vi "FRIC_navX_Internal_USB_ProcessingLoop.vi"(7 "Device Number":T3, 10 "Serial Port":T2=enum."USB 1", 11 "Rate (4Hz-200Hz)":u8=50 min=4 max=200) -> ()   [LabVIEW 2025]
doc: "This navX VI handles the reading/writing for the navX. All of the good stuff is in here.\nTHIS VI SHOULD NOT BE CALLED BY THE USER!"
uses:
  _TypeDefs/Z900_navX_SerialStreamTypeDef.ctl
  _TypeDefs/FRIC_navX_DeviceNumbersTypeDef.ctl
  <vilib>/Rock Robotics/WPI/SerialPort/WPI_SerialPort.ctl
  _TypeDefs/Z900_navX_ProtocolTypeDef.ctl
  _TypeDefs/FRIC_navX_ProcessingLoopStatesTypeDef_I2C.ctl
  _TypeDefs/FRIC_navX_I2C Process Loop TypeDef.ctl
  _TypeDefs/Z900_navX_DeviceTypeDef.ctl
  _TypeDefs/Z900_navX_NotifyPacketTypeDef.ctl
  _TypeDefs/Z900_navX_ActionTypeDef.ctl
  <vilib>/Rock Robotics/SystemInterfaces/i2clib/i2c_bus.ctl
  _TypeDefs/Z900_navX_IntegrationControlRegisters.ctl
  <vilib>/Rock Robotics/WPI/SPI/WPI_SPIDevRef.ctl
  <vilib>/Rock Robotics/SystemInterfaces/spilib/spi_bus.ctl
  <vilib>/Rock Robotics/WPI/SerialPort/WPI_SerialPortRef.ctl
  <vilib>/Platform/TimedLoop/XDataNode/timing_clust.ctl
  <vilib>/Platform/TimedLoop/XDataNode/nitl_modes.ctl
  <vilib>/Platform/TimedLoop/XDataNode/wakeup.ctl
  <vilib>/Rock Robotics/SystemInterfaces/NetworkCommunication/NetComm_UsageReport_ResourceType.ctl
  <vilib>/Rock Robotics/SystemInterfaces/Utilities/FPGA_UtilitiesRead LocalTime.vi
  <vilib>/Platform/TimedLoop/XDataNode/XDataNode.xnode
  <vilib>/Platform/TimedLoop/XDataNode/XDNodeRunTimeDep.lvlib
panel:
  in  "Tab Control":enum32{"Page 1", "Page 2"}(tab)
  in  "Halt":bool
  out "Connected 2":bool
  out "error":errorcluster
  in  "Stream Type":T1=enum."AHRSAndPositioning"
  out "Loop TIme":i64
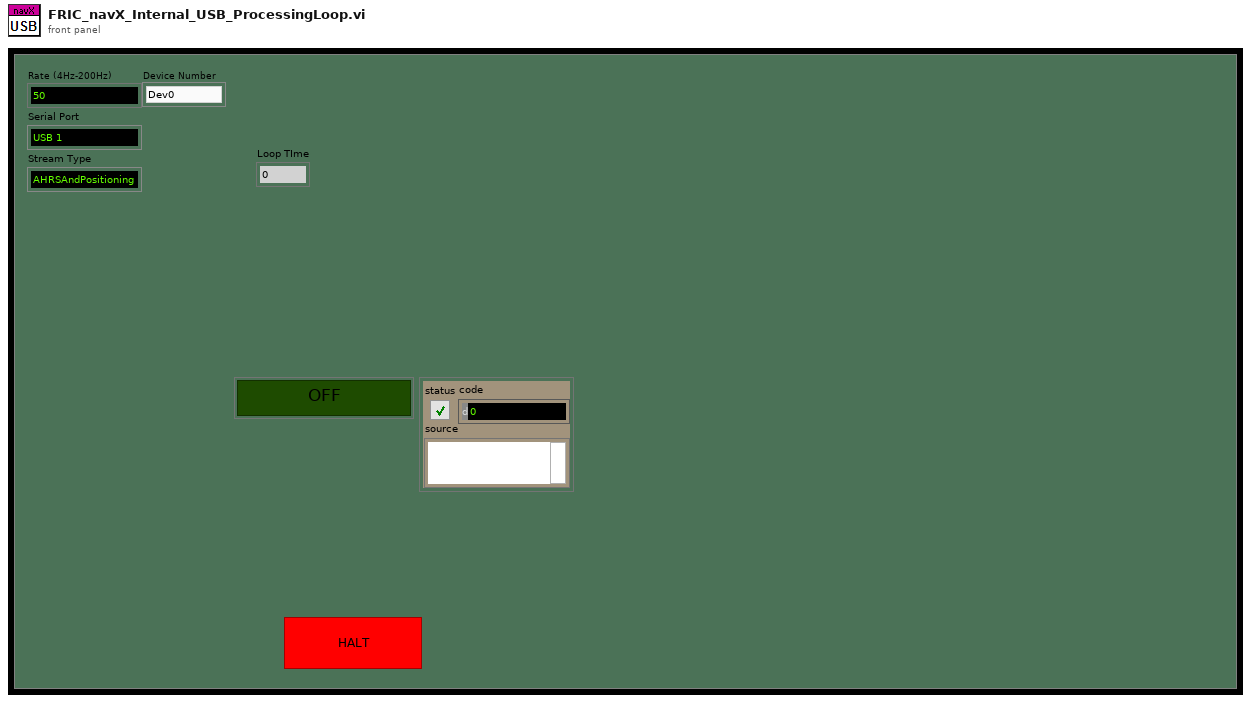
[diagram p1: front panel]
types:
  T1 = typedef "Z900_navX_SerialStreamTypeDef.ctl" = enum16{"YRPH", "Quaterinons", "Gyro/Raw", "AHRS", "AHRSAndPositioning", "AHRSAndPOSTime"}
  T2 = typedef "WPI_SerialPort.ctl" = enum16{"Onboard RS-232", "MXP TTL", "USB 1", "USB 2"}
  T3 = typedef "FRIC_navX_DeviceNumbersTypeDef.ctl" = enum16{"Dev0", "Dev1", "Dev2", "Dev3"}
  T4 = typedef "FRIC_navX_I2C Process Loop TypeDef.ctl" = cluster{"State Array":T5[], "error":errorcluster, "FPGA Cluster":cluster{"Last Valid FPGA Time":dbl, "Error Count":i32, "Initialized":bool}, "Device Info":T6, "I2CDevRef":cluster{"DevStatus":errorcluster, "Device Address":u8, "Handle":i32, "I2C Bus":T8}, "Registry":u8[], "Command Array":T9[], "Connected?":bool, "navX Device Memory Size":i32, "notification":T10, "Memory Size Set":bool, "SPIDevRef":T12, "navX Serial Open":cluster{"Stream Type":T1, "Serial Port":T2}, "SerialPortRef":T14, "Serial Read Buffer":string, "Serial Write Buffer":string[], "Device Number":T3, "navX SPI Open":cluster{"SPI Bus":T13, "Clock Rate (Hz)":dbl}, "Loop dt":i64, "current time":timestamp, "Loop Time":i64}
  T5 = typedef "FRIC_navX_ProcessingLoopStatesTypeDef_I2C.ctl" = enum16{"Process", "INI", "Check Packets Valid", "Close", "Clear VISA", "Generate Command", "Last Packet Valid", "Open", "Read", "Reset Serial", "Set Termination Char", "Update AE", "Wait", "Write", "Exit"}
  T6 = typedef "Z900_navX_DeviceTypeDef.ctl" = cluster{"Interface":cluster{"Protocol":T7, "Update Rate (4Hz-200Hz)":u8, "navX Open TypeDef":variant}, "Notify Packet":refnum<notifier>, "Loop VI Refnum":refnum<vi>, "Ready to Close Occurrence Refnum":refnum<k4>, "Name":string}
  T7 = typedef "Z900_navX_ProtocolTypeDef.ctl" = enum16{"SERIAL", "I2C", "SPI"}
  T8 = typedef "i2c_bus.ctl" = enum16{"I2C On-Board", "I2C MXP", "Invalid"}
  T9 = typedef "Z900_navX_IntegrationControlRegisters.ctl" = u8
  T10 = typedef "Z900_navX_NotifyPacketTypeDef.ctl" = cluster{"navX Action":T11, "Data":variant, "Stream Type":T1, "Device Number":T3}
  T11 = typedef "Z900_navX_ActionTypeDef.ctl" = enum16{"None", "Halt", "Normal Read", "Update Serial Protocol", "Update Rate Htz", "Zero-Yaw", "Zero-Displacement", "Zero-Velocity"}
  T12 = typedef "WPI_SPIDevRef.ctl" = cluster{"DevStatus":errorcluster, "Handle":i32, "SPI Bus":T13}
  T13 = typedef "spi_bus.ctl" = enum16{"SPI On-Board, CS0", "SPI On-Board, CS1", "SPI On-Board, CS2", "SPI On-Board, CS3", "SPI MXP", "Invalid"}
  T14 = typedef "WPI_SerialPortRef.ctl" = cluster{"DevStatus":errorcluster, "Serial Port Name":refnum<visa-resource-name>}
  T15 = typedef "XDNodeRunTimeDep.lvlib/timing_clust.ctl" = cluster{"Expected End [f-1]":u64, "Actual End [f-1]":u64, "Finished Late? [f-1]":bool, "Expected End [i-1]":u64, "Actual End [i-1]":u64, "Finished Late? [i-1]":bool, "Expected Start [i]":u64, "Actual Start [i]":u64, "Expected Start [f]":u64, "Actual Start [f]":u64, "Source Name":string, "Structure Name":string, "Period":i64, "Deadline":i64, "Offset":i64, "Start":i64, "Priority":i32, "Timeout":i32, "Mode":T16, "Wakeup Reason":T17, "Error":errorcluster, "Source Type":string, "Secondary Source Type":string, "Global End Time":u64, "Global Start Time":u64, "Frame Duration":u64, "Iteration Duration":u64, "Assigned CPU":i32, "I/O Scan Engine Mode":u32}
  T16 = typedef "XDNodeRunTimeDep.lvlib/nitl_modes.ctl" = enum32{"No Change", "Process missed periods, maintain original phase", "Discard missed periods, maintain original phase", "Process missed periods, ignore original phase", "Discard missed periods, ignore original phase"}
  T17 = typedef "XDNodeRunTimeDep.lvlib/wakeup.ctl" = enum32{"Normal", "Aborted", "Asynchronous wakeup", "Timing source error", "Timed loop error", "Timeout"}
  T18 = typedef "NetComm_UsageReport_ResourceType.ctl" = enum8{"Controller", "Module", "Language", "CANPlugin", "Accelerometer", "ADXL345", "AnalogChannel", "AnalogTrigger", "AnalogTriggerOutput", "CANJaguar", "Compressor", "Counter", "Dashboard", "DigitalInput", "DigitalOutput", "DriverStationCIO", "DriverStationEIO", "DriverStationLCD", "Encoder", "GearTooth", "Gyro", "I2C", "Framework", "Jaguar", "Joystick", "Kinect", "KinectStick", "PIDController", "Preferences", "PWM", "Relay", "RobotDrive", "SerialPort", "Servo", "Solenoid", "SPI", "Task", "Ultrasonic", "Victor", "Button", "Command", "AxisCamera", "PCVideoServer", "SmartDashboard", "Talon", "HiTechnicColorSensor", "HiTechnicAccel", "HiTechnicCompass", "SRF08", "AnalogOutput", "Victor SP", "Talon SRX", "CAN Talon SRX", "ADXL362 Accel", "ADXRS450 Gyro", "Rev SPARK", "Mindsensors SD540", "Digital Filter", "ADIS16448", "PDP", "PCM", "PigeonIMU", "Nidec Brushless", "CTRE CANifier", "CTRE TalonFX", "CTRE Future 1", "CTRE Future 2", "CTRE Future 3", "CTRE Future 4", "CTRE Future 5", "CTRE Future 6", "Linear Filter", "Xbox Controller", "USB Camera", "NavX", "Pixy", "Pixy2", "ScanseSweep", "Shuffleboard", "CAN", "Digilent DMC60", "PWM Victor SPX", "Rev SPARK MAX PWM", "Rev SPARK MAX CAN", "ADIS16470", "PIDController2", "ProfiledPIDController", "Kinematics", "Odometry", "Units", "Trapezoid Profile", "DutyCycle", "Addressable LEDs", "Fusion Venom", "CTRE Future 7", "CTRE Future 8", "CTRE Future 9", "CTRE Future 10", "CTRE Future 11", "CTRE Future 12", "CTRE Future 13", "CTRE Future 14", "Exponential Profile", "PS4 Controller", "Photon Camera", "Photon Pose Estimator", "Path Planner Path", "Path Planner Auto", "Path Finding Command", "Redux Future 1", "Redux Future 2", "Redux Future 3", "Redux Future 4", "Redux Future 5", "Rev SPARK Flex CAN", "Rev SPARK Flex PWM", "LEDPattern", "LinearQuadraticRegulator", "KalmanFilter", "PoseEstimator", "PoseEstimator3d", "LinearSystemLoop", "WPILib_future7", "WPILib_future8", "Rev_ServoHub", "YAMS", "LumenLabs_ConnectorX", "LumenLabs_ConnectorXLED"}
  T19 = cluster{"Last Valid FPGA Time":dbl, "Error Count":i32, "Initialized":bool}
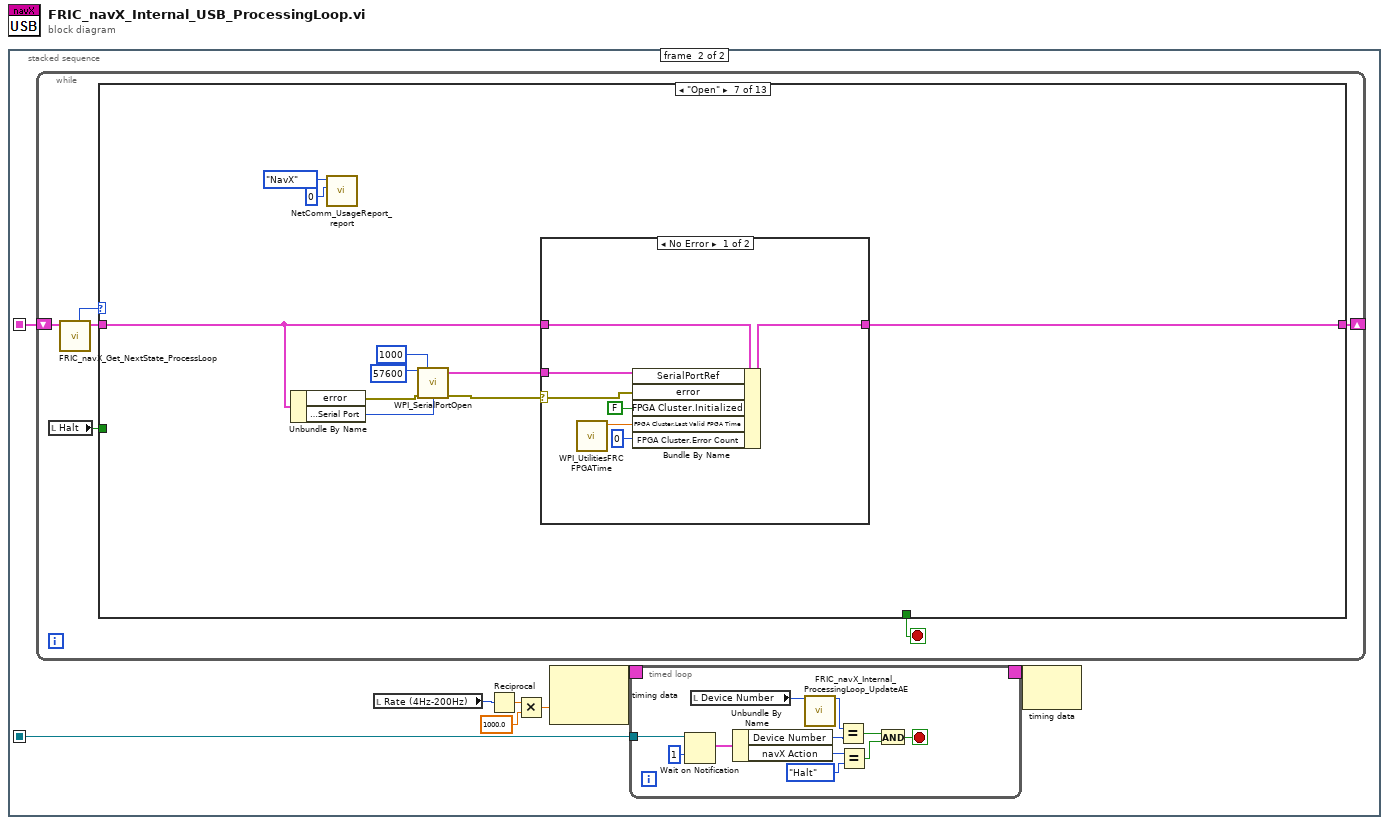
[diagram p0: block diagram]
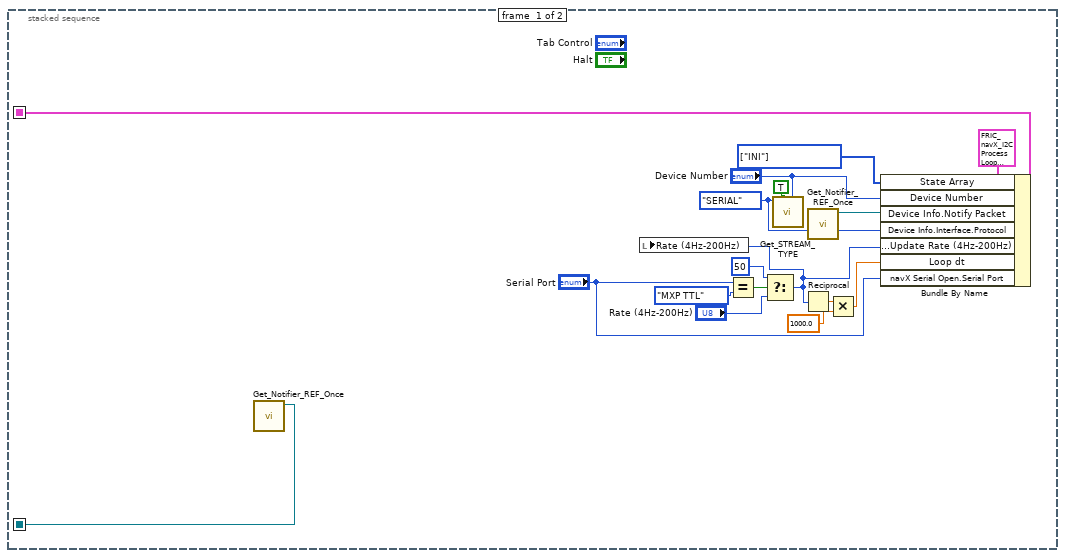
[diagram p2: hidden frame]
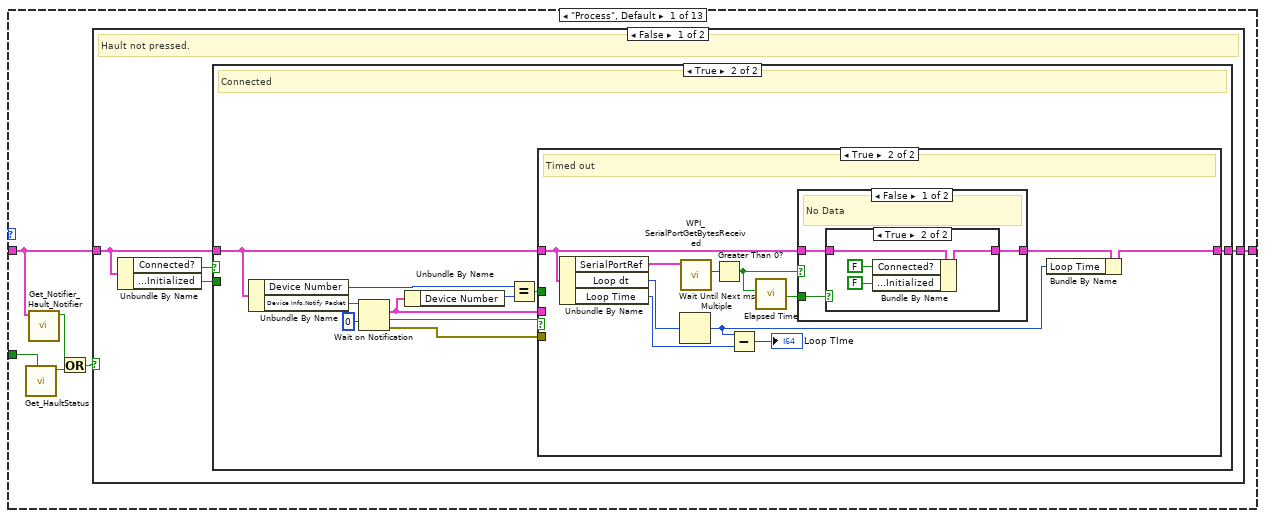
[diagram p3: hidden frame]
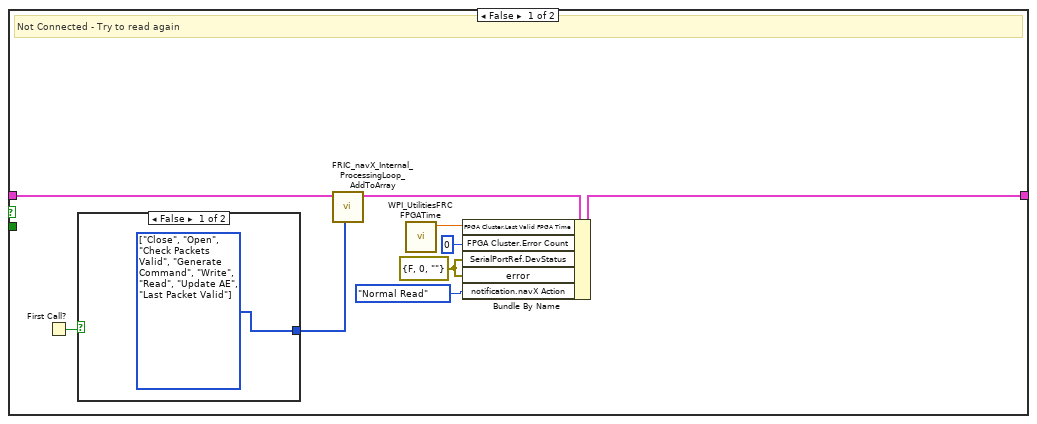
[diagram p4: hidden frame]
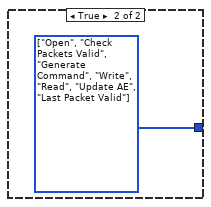
[diagram p5: hidden frame]
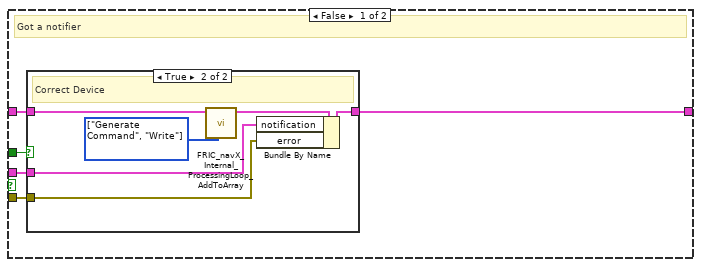
[diagram p6: hidden frame]
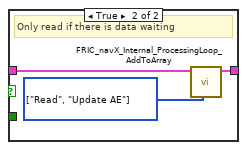
[diagram p9: hidden frame]
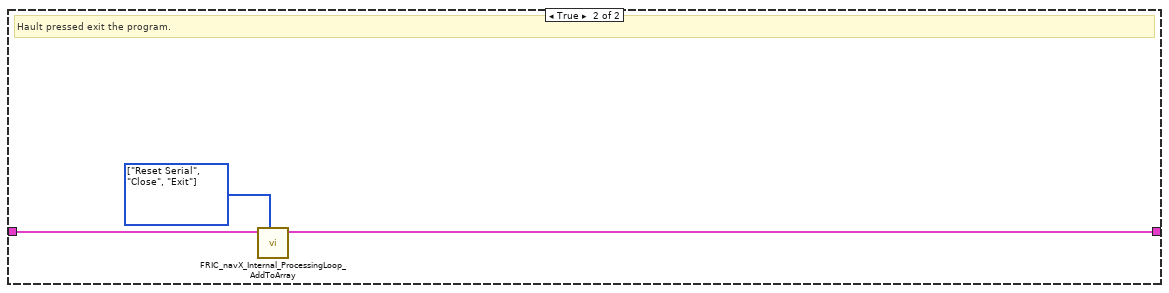
[diagram p10: hidden frame]
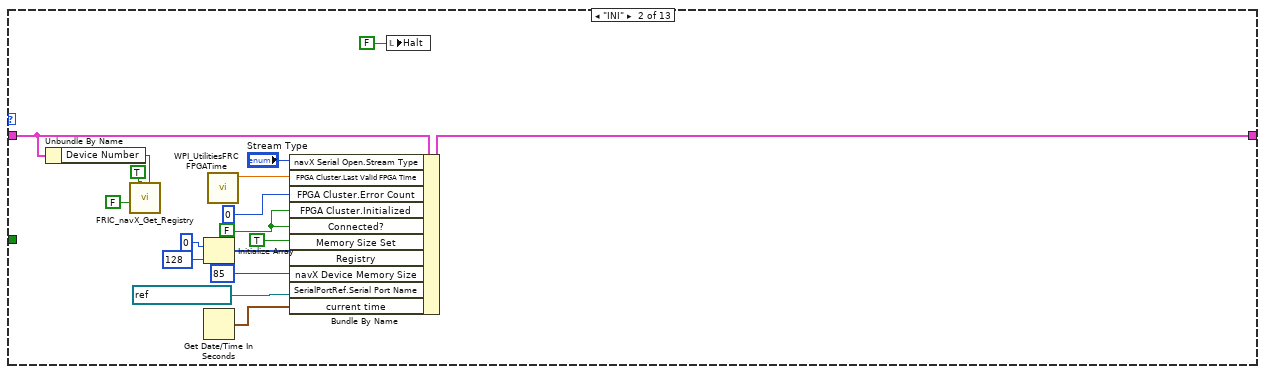
[diagram p11: hidden frame]
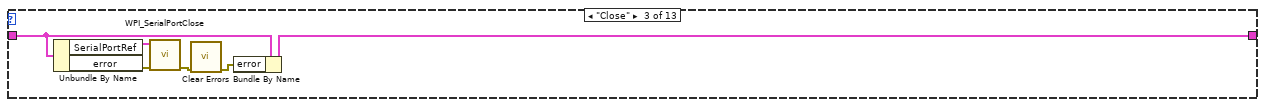
[diagram p12: hidden frame]
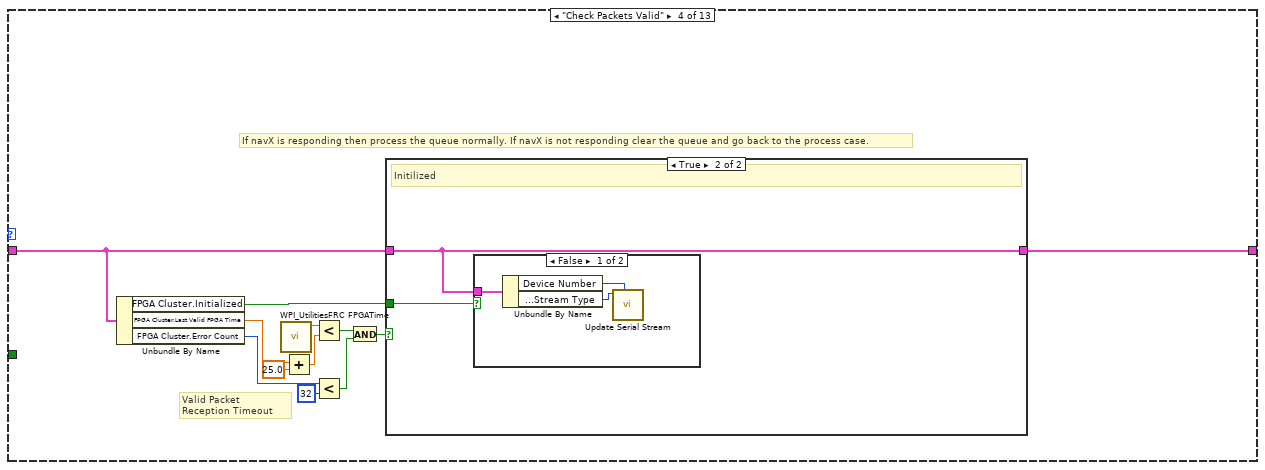
[diagram p13: hidden frame]
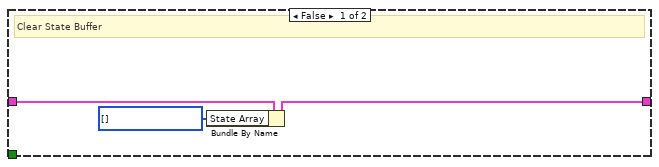
[diagram p14: hidden frame]
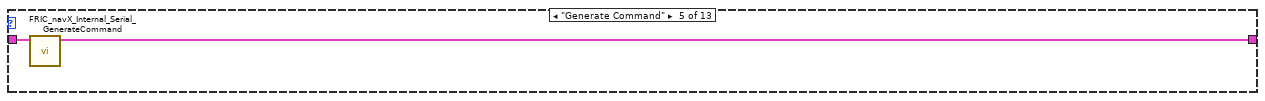
[diagram p16: hidden frame]
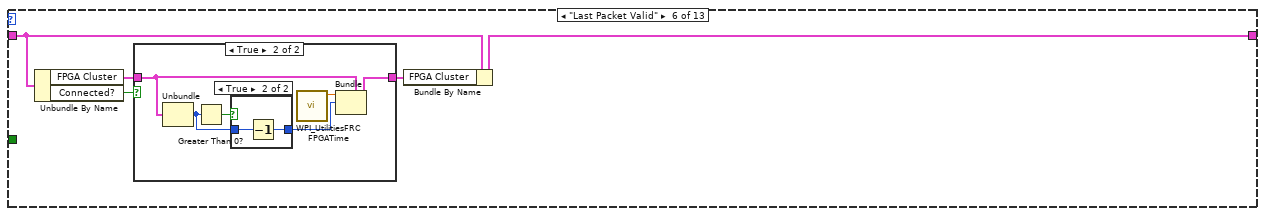
[diagram p17: hidden frame]
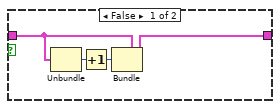
[diagram p18: hidden frame]
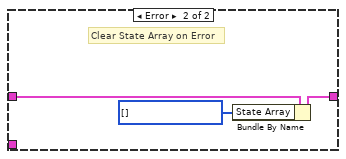
[diagram p20: hidden frame]
diagram:
  n1 = stacked-sequence {
    seq-local: [w17 _] -> [_ w25]
    seq-local: [w13 _] -> [_ w18]
    frame #0 {
      w1 = Z900_navX_ProtocolTypeDef."SERIAL" ("Protocol")
      w15 = T5[] [enum."INI"] items=["Process", "INI", "Check Packets Valid", "Close", "Clear VISA", "Generate Command", "Last Packet Valid", "Open", "Read", "Reset Serial", "Set Termination Char", "Update AE", "Wait", "Write", "Exit"] ("State Array")
      n2 = call "Get_Notifier_REF_Once.vi"() -> ("notifier ref out"=w13:refnum<notifier>)  [unwired: 10 in, 1 out]
      n3 = Equal?(x="Serial Port", y=WPI_SerialPort."MXP TTL") -> (x = y?=w9:bool)
      n4 = Select(t=u8 50, s=w9, f="Rate (4Hz-200Hz)") -> (s? t:f=w4:u8)
      n5 = local write "Rate (4Hz-200Hz)"(w4) -> ()
      n6 = call "Get_STREAM_TYPE.vi"("Device Number"="Device Number", "Update"=TRUE, "Protocol (in)"=w1) -> ()  [unwired: 8 in, 1 out]
      n7 = Reciprocal(x=w4) -> (1/x=w11:dbl)
      n8 = call "Get_Notifier_REF_Once.vi"() -> ("notifier ref out"=w14:refnum<notifier>)  [unwired: 10 in, 1 out]
      n9 = Multiply(x=w11, y=1000.0) -> (x*y=w6:dbl)
      n10 = Bundle By Name(cluster=T4 {"State Array"=[enum."INI", enum."Open"], "error"={"status"=FALSE, "code"=0, "source"=""}, "FPGA Cluster"={"Last Valid FPGA Time"=0.0, "Error Count"=0, "Initialized"=FALSE}, "Device Info"={"Interface"={"Protocol"=enum."SERIAL", "Update Rate (4Hz-200Hz)"=4, "navX Open TypeDef"=variant}, "Notify Packet"=refnum, "Loop VI Refnum"=refnum, "Ready to Close Occurrence Refnum"=refnum, "Name"=""}, "I2CDevRef"={"DevStatus"={"status"=FALSE, "code"=0, "source"=""}, "Device Address"=0, "Handle"=0, "I2C Bus"=enum."Invalid"}, "Registry"=[], "Command Array"=[214, 32], "Connected?"=FALSE, "navX Device Memory Size"=85, "notification"={"navX Action"=enum."None", "Data"=variant, "Stream Type"=enum."YRPH", "Device Number"=enum."Dev0"}, "Memory Size Set"=FALSE, "SPIDevRef"={"DevStatus"={"status"=FALSE, "code"=0, "source"=""}, "Handle"=0, "SPI Bus"=enum."SPI On-Board, CS0"}, "navX Serial Open"={"Stream Type"=enum."YRPH", "Serial Port"=enum."Onboard RS-232"}, "SerialPortRef"={"DevStatus"={"status"=FALSE, "code"=0, "source"=""}, "Serial Port Name"=""}, "Serial Read Buffer"="", "Serial Write Buffer"=[], "Device Number"=enum."Dev0", "navX SPI Open"={"SPI Bus"=enum."SPI MXP", "Clock Rate (Hz)"=500000.0}, "Loop dt"=0, "current time"=timestamp(0 s since 1904-01-01), "Loop Time"=0} ("I2C Process Loop TypeDef"), "State Array"=w15, "Device Number"="Device Number", "Device Info.Notify Packet"=w14, "Device Info.Interface.Protocol"=w1, "Device Info.Interface.Update Rate (4Hz-200Hz)"=w4, "Loop dt"=w6, "navX Serial Open.Serial Port"="Serial Port") -> (w17:T4)
    }
    frame #1 {
      n11 = while {
        shift-right: [w43] -> _
        shift-left: w25 -> [w46]
        stop <- w47 stop-if-true
        n12 = local read "Halt"() -> (w42:bool)
        n13 = call "FRIC_navX_Get_NextState_ProcessLoop.vi"("I2C Process Loop TypeDef (in)"=w46) -> ("I2C Process Loop TypeDef (out)"=w45:T4, "Current State"=w44:T5)  [unwired: 9 in]
        n14 = case shown="\"Open\"" w44 {
          tunnel: [_ _ _ _ _ _ _ _ _ _ TRUE _ _] -> w47
          tunnel: w45 -> [w51 w121 w138 w143 w160 w164 w188 w210 w228 w241 w248 w256 w257]
          tunnel: [w53 w128 w137 w144 w159 w163 w187 w207 w229 w239 w248 w256 w257] -> w43
          tunnel: w42 -> [w52 _ _ _ _ _ _ _ _ _ _ _ _]
          frame "Process", Default {
            n15 = call "Get_HaultStatus.vi"("Update"=w52) -> ("Hault"=w49:bool)  [unwired: 10 in]
            n16 = call "Get_Notifier_Hault_Notifier.vi"("Process Loop TypeDef (in)"=w51) -> ("Hault Notifier"=w50:bool)  [unwired: 10 in]
            n17 = Or(x=w50, y=w49) -> (x .or. y?=w48:bool)
            n18 = case shown="False" w48 {
              tunnel: [w57 w114] -> w53
              tunnel: w51 -> [w55 w115]
              frame False {
                # "Hault not pressed."
                n19 = Unbundle By Name(w55) -> ("Connected?"=w56:bool, "FPGA Cluster.Initialized"=w54:bool)
                n20 = case shown="True" w56 {
                  tunnel: w55 -> [w66 w69]
                  tunnel: [w63 w78] -> w57
                  tunnel: w54 -> [_ _]
                  frame False {
                    w60 = errorcluster {"status"=FALSE, "code"=0, "source"=""} ("SerialPortRef.DevStatus")
                    # "Not Connected - Try to read again"
                    n21 = First Call?() -> (First Call?: T/F=w59:bool)
                    n22 = case shown="False" w59 {
                      tunnel: [w67 w68] -> w65
                      frame False {
                        w67 = T5[] [enum."Close", enum."Open", enum."Check Packets Valid", enum."Generate Command", enum."Write", enum."Read", enum."Update AE", enum."Last Packet Valid"] items=["Process", "INI", "Check Packets Valid", "Close", "Clear VISA", "Generate Command", "Last Packet Valid", "Open", "Read", "Reset Serial", "Set Termination Char", "Update AE", "Wait", "Write", "Exit"]
                      }
                      frame True {
                        w68 = T5[] [enum."Open", enum."Check Packets Valid", enum."Generate Command", enum."Write", enum."Read", enum."Update AE", enum."Last Packet Valid"] items=["Process", "INI", "Check Packets Valid", "Close", "Clear VISA", "Generate Command", "Last Packet Valid", "Open", "Read", "Reset Serial", "Set Termination Char", "Update AE", "Wait", "Write", "Exit"]
                      }
                    }
                    n23 = call "FRIC_navX_Internal_ProcessingLoop_AddToArray.vi"("States Array"=w65, "I2C Process Loop TypeDef (in)"=w66) -> ("I2C Process Loop TypeDef (out)"=w64:T4)  [unwired: 9 in]
                    n24 = call <vilib>:"WPI_UtilitiesFRC FPGATime.vi"() -> ("FPGA Time"=w61:dbl)  [unwired: 10 in, 1 out]
                    n25 = Bundle By Name(cluster=w64, "FPGA Cluster.Last Valid FPGA Time"=w61, "FPGA Cluster.Error Count"=0, "SerialPortRef.DevStatus"=w60, "error"=w60, "notification.navX Action"=Z900_navX_ActionTypeDef."Normal Read") -> (w63:T4)
                  }
                  frame True {
                    # "Connected"
                    n26 = Unbundle By Name(w69) -> ("Device Number"=w72:T3, "Device Info.Notify Packet"=w77:refnum<notifier>)
                    n27 = Wait on Notification(notifier=w77, timeout in ms (-1)=0) -> (notification=w73:T10, timed out?=w74:bool, error out=w75:errorcluster)  [unwired: 2 in, 1 out]
                    n28 = Unbundle By Name(w73) -> ("Device Number"=w71:T3)
                    n29 = Equal?(x=w72, y=w71) -> (x = y?=w70:bool)
                    n30 = case shown="True" w74 {
                      tunnel: w69 -> [w83 w99]
                      tunnel: [w82 w94] -> w78
                      tunnel: w73 -> [w81 _]
                      tunnel: w75 -> [w80 _]
                      tunnel: w70 -> [w79 _]
                      frame False {
                        # "Got a notifier"
                        n31 = case shown="True" w79 {
                          tunnel: w83 -> [w84 w90]
                          tunnel: [w84 w89] -> w82
                          tunnel: w81 -> [_ w88]
                          tunnel: w80 -> [_ w85]
                          frame False {
                          }
                          frame True {
                            w86 = T5[] [enum."Generate Command", enum."Write"] items=["Process", "INI", "Check Packets Valid", "Close", "Clear VISA", "Generate Command", "Last Packet Valid", "Open", "Read", "Reset Serial", "Set Termination Char", "Update AE", "Wait", "Write", "Exit"] ("States Array")
                            # "Correct Device"
                            n32 = call "FRIC_navX_Internal_ProcessingLoop_AddToArray.vi"("States Array"=w86, "I2C Process Loop TypeDef (in)"=w90) -> ("I2C Process Loop TypeDef (out)"=w87:T4)  [unwired: 9 in]
                            n33 = Bundle By Name(cluster=w87, "notification"=w88, "error"=w85) -> (w89:T4)
                          }
                        }
                      }
                      frame True {
                        # "Timed out"
                        n34 = Unbundle By Name(w99) -> ("SerialPortRef"=w101:T14, "Loop dt"=w96:i64, "Loop Time"=w92:i64)
                        n35 = Wait Until Next ms Multiple(millisecond multiple=w96) -> (millisecond timer value=w93:u32)
                        n36 = call <vilib>:"WPI_SerialPortGetBytesReceived.vi"("SerialPortRef"=w101) -> ("Bytes at Port"=w100:u32)  [unwired: 8 in, 2 out]
                        n37 = Greater Than 0?(x=w100) -> (x > 0?=w98:bool)
                        n38 = Subtract(x=w93, y=w92) -> (x-y=→"Loop TIme":i64)
                        n39 = call "Elapsed Time"("Reset"=w98) -> ("Time has Elapsed"=w97:bool)  [unwired: 11 in, 7 out]
                        n40 = case shown="False" w98 {
                          tunnel: [w103 w111] -> w95
                          tunnel: w99 -> [w104 w110]
                          tunnel: w97 -> [w102 _]
                          frame False {
                            # "No Data"
                            n41 = case shown="True" w102 {
                              tunnel: w104 -> [w105 w109]
                              tunnel: [w105 w108] -> w103
                              frame False {
                              }
                              frame True {
                                n42 = Bundle By Name(cluster=w109, "Connected?"=FALSE, "FPGA Cluster.Initialized"=FALSE) -> (w108:T4)
                              }
                            }
                          }
                          frame True {
                            w112 = T5[] [enum."Read", enum."Update AE"] items=["Process", "INI", "Check Packets Valid", "Close", "Clear VISA", "Generate Command", "Last Packet Valid", "Open", "Read", "Reset Serial", "Set Termination Char", "Update AE", "Wait", "Write", "Exit"]
                            # "Only read if there is data waiting"
                            n43 = call "FRIC_navX_Internal_ProcessingLoop_AddToArray.vi"("States Array"=w112, "I2C Process Loop TypeDef (in)"=w110) -> ("I2C Process Loop TypeDef (out)"=w111:T4)  [unwired: 9 in]
                          }
                        }
                        n44 = Bundle By Name(cluster=w95, "Loop Time"=w93) -> (w94:T4)
                      }
                    }
                  }
                }
              }
              frame True {
                w113 = T5[] [enum."Reset Serial", enum."Close", enum."Exit"] items=["Process", "INI", "Check Packets Valid", "Close", "Clear VISA", "Generate Command", "Last Packet Valid", "Open", "Read", "Reset Serial", "Set Termination Char", "Update AE", "Wait", "Write", "Exit"] ("States Array")
                # "Hault pressed exit the program."
                n45 = call "FRIC_navX_Internal_ProcessingLoop_AddToArray.vi"("States Array"=w113, "I2C Process Loop TypeDef (in)"=w115) -> ("I2C Process Loop TypeDef (out)"=w114:T4)  [unwired: 9 in]
              }
            }
          }
          frame "INI" {
            w126 = FALSE ("Initialized")
            n46 = Unbundle By Name(w121) -> ("Device Number"=w120:T3)
            n47 = call "FRIC_navX_Get_Registry.vi"("Device Number"=w120, "Update"=TRUE, "Connected?"=FALSE) -> ()  [unwired: 7 in, 2 out]
            n48 = Initialize Array(u8 0 ("Received Data"), 128 ("hex")) -> (w124:u8[])
            n49 = Get Date/Time In Seconds() -> (seconds since 1Jan1904=w116:timestamp)
            n50 = call <vilib>:"WPI_UtilitiesFRC FPGATime.vi"() -> ("FPGA Time"=w130:dbl)  [unwired: 10 in, 1 out]
            n51 = Bundle By Name(cluster=w121, "navX Serial Open.Stream Type"="Stream Type", "FPGA Cluster.Last Valid FPGA Time"=w130, "FPGA Cluster.Error Count"=0 ("Error Count"), "FPGA Cluster.Initialized"=w126, "Connected?"=w126, "Memory Size Set"=TRUE, "Registry"=w124, "navX Device Memory Size"=85 ("hex"), "SerialPortRef.Serial Port Name"=refnum<visa-resource-name> "ASRL3::INSTR" ("Serial Port Name"), "current time"=w116) -> (w128:T4)
            n52 = local write "Halt"(FALSE ("Halt")) -> ()
          }
          frame "Close" {
            n53 = Unbundle By Name(w138) -> ("SerialPortRef"=w135:T14, "error"=w134:errorcluster)
            n54 = call <vilib>:"WPI_SerialPortClose.vi"("error in (no error)"=w134, "SerialPortRef"=w135) -> ("error out"=w133:errorcluster)  [unwired: 9 in]
            n55 = call <vilib>:"Clear Errors.vi"("error in (no error)"=w133) -> ("error out"=w136:errorcluster)  [unwired: 5 in, 1 out]
            n56 = Bundle By Name(cluster=w138, "error"=w136) -> (w137:T4)
          }
          frame "Check Packets Valid" {
            # "If navX is responding then process the queue normally. If navX is not responding clear the queue and go back to the process case."
            # "Valid Packet Reception Timeout"
            n57 = Unbundle By Name(w143) -> ("FPGA Cluster.Initialized"=w139:bool, "FPGA Cluster.Last Valid FPGA Time"=w142:dbl, "FPGA Cluster.Error Count"=w141:i32)
            n58 = call <vilib>:"WPI_UtilitiesFRC FPGATime.vi"() -> ("FPGA Time"=w148:dbl)  [unwired: 10 in, 1 out]
            n59 = Add(x=w142, y=25.0) -> (x+y=w149:dbl)
            n60 = Less?(x=w148, y=w149) -> (x < y?=w146:bool)
            n61 = Less?(x=w141, y=32) -> (x < y?=w145:bool)
            n62 = And(x=w146, y=w145) -> (x .and. y?=w140:bool)
            n63 = case shown="True" w140 {
              tunnel: w143 -> [w153 w155]
              tunnel: [w152 w155] -> w144
              tunnel: w139 -> [_ w154]
              frame False {
                w151 = T5[] [] items=["Process", "INI", "Check Packets Valid", "Close", "Clear VISA", "Generate Command", "Last Packet Valid", "Open", "Read", "Reset Serial", "Set Termination Char", "Update AE", "Wait", "Write", "Exit"] ("f")
                # "Clear State Buffer"
                n64 = Bundle By Name(cluster=w153, "State Array"=w151) -> (w152:T4)
              }
              frame True {
                # "Initilized"
                n65 = case shown="False" w154 {
                  tunnel: w155 -> [w156 _]
                  frame False {
                    n66 = Unbundle By Name(w156) -> ("Device Number"=w157:T3, "navX Serial Open.Stream Type"=w158:T1)
                    n67 = call "Update Serial Stream.vi"("Device Number"=w157, "Stream Type"=w158) -> ()  [unwired: 10 in]
                  }
                  frame True {
                  }
                }
              }
            }
          }
          frame "Generate Command" {
            n68 = call "FRIC_navX_Internal_Serial_GenerateCommand.vi"("Serial Process Loop TypeDef (in)"=w160) -> ("Serial Process Loop TypeDef (out)"=w159:T4)  [unwired: 10 in]
          }
          frame "Last Packet Valid" {
            n69 = Unbundle By Name(w164) -> ("FPGA Cluster"=w165:T19, "Connected?"=w161:bool)
            n70 = case shown="True" w161 {
              tunnel: [w168 w175] -> w162
              tunnel: w165 -> [w167 w171]
              frame False {
                n71 = Unbundle(w167) -> ("Error Count"=w166:i32)  [unwired: 2 out]
                n72 = Increment(x=w166) -> (x+1=w169:i32)
                n73 = Bundle(cluster=w167, "Error Count"=w169) -> (w168:T19)  [unwired: 2 in]
              }
              frame True {
                n74 = Unbundle(w171) -> ("Error Count"=w170:i32)  [unwired: 2 out]
                n75 = Greater Than 0?(x=w170) -> (x > 0?=w173:bool)
                n76 = case shown="True" w173 {
                  tunnel: [w176 w178] -> w172
                  tunnel: w170 -> [w176 w177]
                  frame False {
                  }
                  frame True {
                    n77 = Decrement(x=w177) -> (x-1=w178:i32)
                  }
                }
                n78 = call <vilib>:"WPI_UtilitiesFRC FPGATime.vi"() -> ("FPGA Time"=w174:dbl)  [unwired: 10 in, 1 out]
                n79 = Bundle(cluster=w171, "Last Valid FPGA Time"=w174, "Error Count"=w172) -> (w175:T19)  [unwired: 1 in]
              }
            }
            n80 = Bundle By Name(cluster=w164, "FPGA Cluster"=w162) -> (w163:T4)
          }
          frame "Open" {
            n81 = Unbundle By Name(w188) -> ("error"=w184:errorcluster, "navX Serial Open.Serial Port"=w182:T2)
            n82 = call <vilib>:"NetComm_UsageReport_report.vi"("Instance Number"=u8 0, "Resource Type"=NetComm_UsageReport_ResourceType."NavX") -> ()  [unwired: 10 in]
            n83 = call <vilib>:"WPI_SerialPortOpen.vi"("Baud Rate"=u32 57600, "Timeout Value (ms)"=u32 1000, "error in (no error)"=w184, "Serial Port"=w182) -> ("SerialPortRef"=w186:T14, "error out"=w185:errorcluster)  [unwired: 10 in]
            n84 = case shown="No Error" w185 {
              selector: w185 -> [w190 _]
              tunnel: w188 -> [w189 w196]
              tunnel: [w195 w198] -> w187
              tunnel: w186 -> [w193 _]
              frame No Error {
                n85 = call <vilib>:"WPI_UtilitiesFRC FPGATime.vi"() -> ("FPGA Time"=w192:dbl)  [unwired: 10 in, 1 out]
                n86 = Bundle By Name(cluster=w189, "SerialPortRef"=w193, "error"=w190, "FPGA Cluster.Initialized"=FALSE ("Initialized"), "FPGA Cluster.Last Valid FPGA Time"=w192, "FPGA Cluster.Error Count"=0) -> (w195:T4)
              }
              frame Error {
                w197 = T5[] [] items=["Process", "INI", "Check Packets Valid", "Close", "Clear VISA", "Generate Command", "Last Packet Valid", "Open", "Read", "Reset Serial", "Set Termination Char", "Update AE", "Wait", "Write", "Exit"] ("State Array")
                # "Clear State Array on Error"
                n87 = Bundle By Name(cluster=w196, "State Array"=w197) -> (w198:T4)
              }
            }
          }
          frame "Read" {
            n88 = Unbundle By Name(w210) -> ("Serial Read Buffer"=w213:string, "SerialPortRef"=w214:T14, "SerialPortRef.Serial Port Name"=w216:refnum<visa-resource-name>, "error"=w215:errorcluster, "Device Number"=w206:T3, "Registry"=w211:u8[])
            n89 = property class="Instr"(reference=w216, error in=w215) -> (error out=w212:errorcluster, "Bytes at Port"=w199:u32)  [unwired: 1 in]
            n90 = call <vilib>:"WPI_SerialPortRead.vi"("error in (no error)"=w212, "Num Bytes to Read"=w199, "SerialPortRef"=w214) -> ("error out"=w205:errorcluster, "Buffer"=w203:string)  [unwired: 6 in, 1 out]
            n91 = call "FRIC_navX_Clear_Buffer_Warning.vi"("error in"=w205) -> ("error out"=w204:errorcluster)  [unwired: 10 in]
            n92 = Concatenate Strings(w213, w203) -> (w209:string)
            n93 = Not(x=w204) -> (.not. x?=w200:bool)
            "Connected 2" <- w200
            n94 = call "Z900_navX_SERIAL_CapturePacket.vi"("Buffer"=w209) -> ("Packet Located"=w201:bool, "Packet"=w202:string, "Buffer"=w208:string)  [unwired: 7 in, 1 out]
            n95 = Bundle By Name(cluster=w210, "Serial Read Buffer"=w208, "Connected?"=w200, "error"=w204) -> (w207:T4)
            n96 = case shown="True" w201 {
              tunnel: w211 -> [_ w223]
              tunnel: w200 -> [_ w220]
              tunnel: w206 -> [_ w219]
              tunnel: w202 -> [_ w218]
              frame False {
              }
              frame True {
                n97 = call "Z900_navX_SERIAL_DecodePacket.vi"("Data (in)"=w223, "Packet (in)"=w218) -> ("Data"=w222:u8[])  [unwired: 7 in, 2 out]
                n98 = call "FRIC_navX_Get_Registry.vi"("Device Number"=w219, "Update"=TRUE, "Connected?"=w220, "Registry (in)"=w222) -> ()  [unwired: 6 in, 2 out]
                n99 = call "Get_Connect_Status.vi"("Device Number"=w219, "Update"=TRUE, "Connected"=w220) -> ()  [unwired: 8 in, 1 out]
              }
            }
          }
          frame "Reset Serial" {
            n100 = Unbundle By Name(w228) -> ("SerialPortRef"=w227:T14, "error"=w225:errorcluster)
            n101 = call <vilib>:"WPI_SerialPortReset.vi"("error in (no error)"=w225, "SerialPortRef"=w227) -> ("error out"=w224:errorcluster, "SerialPortRef"=w226:T14)  [unwired: 8 in]
            n102 = Bundle By Name(cluster=w228, "SerialPortRef"=w226, "error"=w224) -> (w229:T4)
          }
          frame "Write" {
            n103 = Unbundle By Name(w241) -> ("SerialPortRef"=w231:T14, "Serial Write Buffer"=w240:string[], "SerialPortRef.DevStatus"=w230:errorcluster)
            n104 = Delete From Array(array=w240, index=0) -> (deleted portion=w236:string, array with subset deleted=w233:string[])  [unwired: 1 in]
            n105 = call <vilib>:"WPI_SerialPortWrite.vi"("error in (no error)"=w230, "Buffer"=w236, "SerialPortRef"=w231) -> ("error out"=w238:errorcluster, "SerialPortRef"=w237:T14)  [unwired: 6 in, 1 out]
            n106 = Empty Array?(array=w233) -> (empty?=w232:bool)
            n107 = Bundle By Name(cluster=w241, "SerialPortRef"=w237, "error"=w238, "Serial Write Buffer"=w233) -> (w234:T4)
            n108 = case shown="False" w232 {
              tunnel: [w245 w246] -> w239
              tunnel: w234 -> [w244 w246]
              frame False {
                w243 = T5[] [enum."Write"] items=["Process", "INI", "Check Packets Valid", "Close", "Clear VISA", "Generate Command", "Last Packet Valid", "Open", "Read", "Reset Serial", "Set Termination Char", "Update AE", "Wait", "Write", "Exit"] ("States Array")
                # "Write again because buffer is not empty."
                n109 = call "FRIC_navX_Internal_ProcessingLoop_AddToArray.vi"("Add to beginning"=TRUE, "States Array"=w243, "I2C Process Loop TypeDef (in)"=w244) -> ("I2C Process Loop TypeDef (out)"=w245:T4)  [unwired: 8 in]
              }
              frame True {
                # "Process the rest of the state array"
              }
            }
          }
          frame "Exit" {
            (unwired) TRUE
            n110 = Unbundle By Name(w248) -> ("Device Info"=w247:T6)
            n111 = in-place {
              in-place-border: w247 -> [w251]
              # "Set Occurence of Close"
              n112 = Unbundle By Name(w251) -> ("Ready to Close Occurrence Refnum"=w252:refnum<k4>)
              n113 = local write "Halt"(FALSE ("Halt")) -> ()
              n114 = Set Occurrence(w252) -> ()
            }
          }
          frame "Update AE" {
            n115 = Unbundle By Name(w256) -> ("Device Number"=w253:T3, "error"=w255:errorcluster)
            "error" <- w255
            n116 = call "Get_Error_Status.vi"("Device Number"=w253, "Update"=TRUE, "error in"=w255) -> ()  [unwired: 8 in, 1 out]
          }
          frame "Clear VISA" {
          }
        }
      }
      n117 = local read "Rate (4Hz-200Hz)"() -> (w23:u8)
      n118 = Reciprocal(x=w23) -> (1/x=w24:dbl)
      n119 = Multiply(x=w24, y=1000.0) -> (x*y=w19:dbl)
      n120 = node-c288(w19) -> (w21:T15)  [unwired: 1 in]
      n121 = timed-loop {
        timing: w21 -> [_]
        timing-out: [_] -> w20
        tunnel: w18 -> [w32]
        stop <- w26 stop-if-true
        n122 = Wait on Notification(notifier=w32, timeout in ms (-1)=1) -> (notification=w31:T10)  [unwired: 2 in, 3 out]
        n123 = local read "Device Number"() -> (w29:T3)
        n124 = Unbundle By Name(w31) -> ("Device Number"=w30:T3, "navX Action"=w34:T11)
        n125 = call "FRIC_navX_Internal_ProcessingLoop_UpdateAE.vi"("Device Number"=w29) -> ()  [unwired: 15 in]
        n126 = Equal?(x=w29, y=w30) -> (x = y?=w28:bool)
        n127 = Equal?(x=w34, y=Z900_navX_ActionTypeDef."Halt") -> (x = y?=w27:bool)
        n128 = And(x=w28, y=w27) -> (x .and. y?=w26:bool)
      }
      n129 = node-c288(w20) -> ()  [unwired: 1 out]
    }
  }
